vi "Assert Excel Save.vi"() -> ()   [LabVIEW 2015]
panel:
  out "data":string[][](array[string])
  in  "path":path
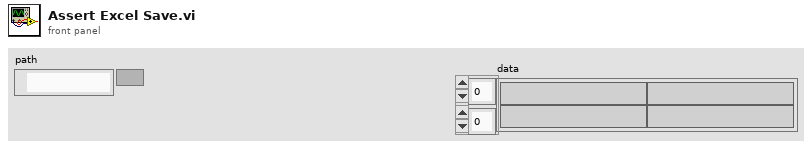
[diagram p1: front panel]
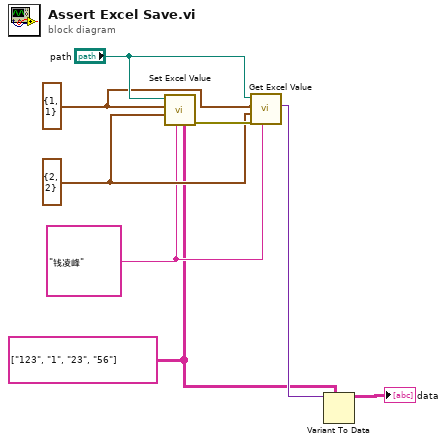
[diagram p0: block diagram]
diagram:
  w2 = string[][] [["123", "1"], ["23", "56"]] ("Excel_Values")
  w4 = "钱凌峰" ("SheetName(\"\")")
  w5 = cluster{"Column":i32, "Row":i32} {"Column"=2, "Row"=2} ("End")
  w6 = cluster{"Column":i32, "Row":i32} {"Column"=1, "Row"=1} ("Start")
  n1 = call "Set Excel Value.vi"("Excel_Values"=w2, "SheetName(\"\")"=w4, "End"=w5, "Start"=w6, "path"="path") -> ("error out"=w8:errorcluster)  [unwired: 6 in]
  n2 = call "Get Excel Value.vi"("SheetName(\"\")"=w4, "error in (no error)"=w8, "End"=w5, "Start"=w6, "path"="path") -> ("Excel_Value"=w3:variant)  [unwired: 5 in, 1 out]
  n3 = Variant To Data(type=w2, Variant=w3) -> (data=→"data":string[][])  [unwired: 1 in, 1 out]
